vi "Host.vi"() -> ()   [LabVIEW 2018]
uses:
  <vilib>/Utility/file.llb/Write Delimited Spreadsheet (I64).vi
  <vilib>/FPGAPlugInAG/PXIe-7976R/niLvFpga_Open_PXIe-7976R.vi
  <vilib>/rvi/interface/common/dynamic/niFpgaDynamicAddResources.vi
  <vilib>/Utility/error.llb/Error Cluster From Error Code.vi
  <vilib>/rvi/errors/niLvFpgaAdjustHostInterfaceError.vi
  <vilib>/rvi/interface/nirviOpenFPGA/nirviOpenFPGA.xnode
  FPGA Bitfiles/Bell-Measurement_FPGATarget_Cluster-Find_279876xpHO0.lvbitx
  BellMeasurement.vi
  <vilib>/rvi/interface/nirviReadWriteControl/nirviReadWriteControl.xnode
  <vilib>/rvi/interface/nirviMethod/nirviMethod.xnode
  NiFpgaLv.dll
  <vilib>/rvi/interface/Simulation/niFpgaSimulationCallBeginRW.vi
  <vilib>/FPGAPlugInAG/Dynamic/niLvFpga_ReadFifo_Dynamic.vi
  <vilib>/rvi/errors/niLvFpgaMergeErrorWithErrorCode.vi
panel:
  in  "Path":path
  in  "stop":bool
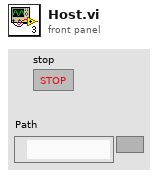
[diagram p1: front panel]
types:
  T1 = enum16{"open", "replace", "create", "open or create", "replace or create", "replace or create with confirmation"}
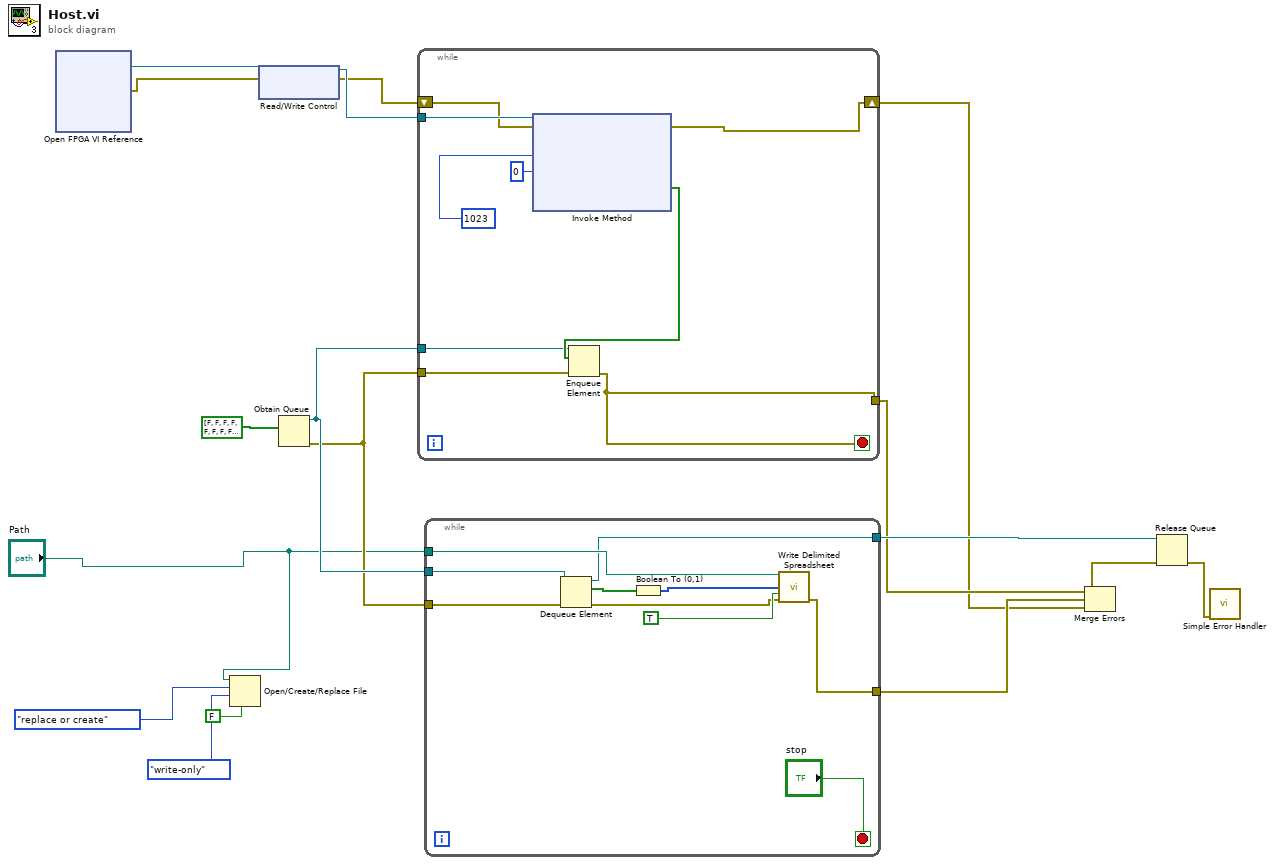
[diagram p0: block diagram]
diagram:
  n1 = xnode "Open FPGA VI Reference"() -> ("FPGA VI Reference Out"=w17:refnum<k20>, "error out"=w16:errorcluster)  [unwired: 2 in]
  n2 = Open/Create/Replace File(file path (use dialog)="Path", operation (0:open)=T1."replace or create", access (0:read/write)=enum16{"read/write", "read-only", "write-only"}."write-only", disable buffering (F)=FALSE) -> ()  [unwired: 2 in, 3 out]
  n3 = xnode "Read/Write Control"("FPGA VI Reference In"=w17, "error in"=w16) -> ("FPGA VI Reference Out"=w15:refnum<k20>, "error out"=w14:errorcluster)  [unwired: 1 out]
  n4 = Obtain Queue(element data type=bool[] [FALSE, FALSE, FALSE, FALSE, FALSE, FALSE, FALSE, FALSE, FALSE, FALSE, FALSE, FALSE, FALSE, FALSE, FALSE, FALSE, FALSE, FALSE, FALSE, FALSE, FALSE, FALSE, FALSE, FALSE, FALSE, FALSE, FALSE, FALSE, FALSE, FALSE, FALSE, FALSE, FALSE, FALSE, FALSE, FALSE, FALSE, FALSE, FALSE, FALSE, FALSE, FALSE, FALSE, FALSE, FALSE, FALSE, FALSE, FALSE, FALSE, FALSE, FALSE, FALSE, FALSE, FALSE, FALSE, FALSE, FALSE, FALSE, FALSE, FALSE, FALSE, FALSE, FALSE, FALSE]) -> (queue out=w12:refnum<queue>, error out=w11:errorcluster)  [unwired: 4 in, 1 out]
  n5 = while {
    tunnel: w15 -> [w26]
    tunnel: w11 -> [w21]
    tunnel: w12 -> [w20]
    shift-right: [w18] -> w3
    shift-left: w14 -> [w25]
    tunnel: [w19] -> w4
    stop <- w19 stop-if-true
    n6 = xnode "Invoke Method"("FPGA VI Reference In"=w26, "error in"=w25, "Number of Elements"=u32 1023, "Timeout (ms)"=0) -> ("error out"=w18:errorcluster, "Data"=w22:bool[])  [unwired: 2 out]
    n7 = Enqueue Element(queue=w20, element=w22, error in (no error)=w21) -> (error out=w19:errorcluster)  [unwired: 1 in, 2 out]
  }
  n8 = while {
    tunnel: w12 -> [w36]
    tunnel: w11 -> [w35]
    tunnel: "Path" -> [w31]
    tunnel: [w29] -> w10
    tunnel: [w28] -> w8
    stop <- "stop" stop-if-true
    n9 = Dequeue Element(queue=w36, error in (no error)=w35) -> (queue out=w28:refnum<queue>, element=w34:bool[], error out=w30:errorcluster)  [unwired: 1 in, 1 out]
    n10 = Boolean To (0,1)(Boolean=w34) -> (0, 1=w33:i16[])
    n11 = call-poly <vilib>:"Write Delimited Spreadsheet.vi"("file path (dialog if empty)"=w31, "1D data"=w33, "append to file? (new file:F)"=TRUE, "error in (no error)"=w30) -> ("error out"=w29:errorcluster)  [unwired: 10 in, 1 out]
  }
  n12 = Merge Errors(w4, w10, w3) -> (w9:errorcluster)
  n13 = Release Queue(queue=w8, error in (no error)=w9) -> (error out=w7:errorcluster)  [unwired: 1 in, 2 out]
  n14 = call <vilib>:"Simple Error Handler.vi"("error in (no error)"=w7) -> ()  [unwired: 4 in, 5 out]
